vi "open vis in library.vi"(8 "error in":errorcluster, 10 "library path":path, 11 "app":refnum<vi>) -> (0 "error out":errorcluster, 2 "vi refs":refnum<vi>[](array[refnum]), 3 "library ref":refnum<vi>)   [LabVIEW 2013, in "scripting tools.lvlib"]
uses:
  scripting tools.lvlib
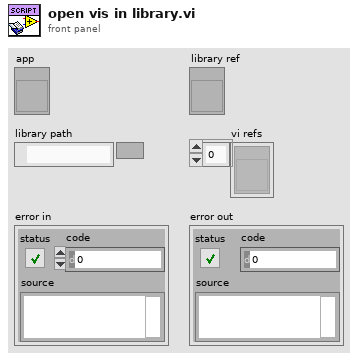
[diagram p1: front panel]
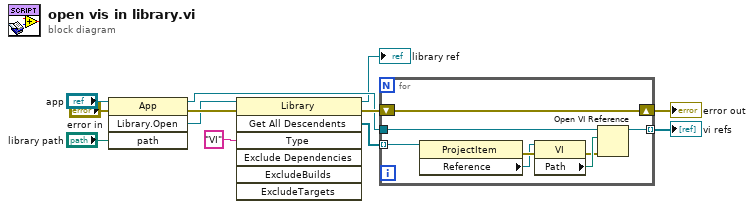
[diagram p0: block diagram]
diagram:
  n1 = invoke class="App" method="Library.Open"(reference="app", error in="error in", "path"="library path") -> (reference out=w8:refnum<vi>, error out=w12:errorcluster, "Open Library"=w11:refnum<vi>)  [unwired: 1 in, 1 out]
  n2 = invoke class="Library" method="Get All Descendents"(reference=w11, error in=w12, "Type"="VI") -> (reference out=→"library ref":refnum<vi>, error out=w9:errorcluster, "All Descendents"=w7:refnum<vi>[])  [unwired: 4 in, 4 out]
  n3 = for {
    tunnel: [w16] -> w6 mode=indexing
    shift-right: [w15] -> w5
    shift-left: w9 -> [w15]
    tunnel: w8 -> [w14]
    tunnel: w7 -> [w13] mode=indexing
    n4 = property class="ProjectItem"(reference=w13) -> (error out=w20:errorcluster, "Reference"=w19:refnum<vi>)  [unwired: 1 in, 1 out]
    n5 = property class="VI"(reference=w19, error in=w20) -> (error out=w17:errorcluster, "Path"=w18:path)  [unwired: 1 out]
    n6 = Open VI Reference(application reference (local)=w14, vi path=w18, error in (no error)=w17) -> (vi reference=w16:refnum<vi>)  [unwired: 3 in, 1 out]
  }
  "vi refs" <- w6
  "error out" <- w5
